vi "Current Loop 9505 (FPGA).vi"() -> ()   [LabVIEW 2011]
uses:
  <vilib>/LabVIEW Targets/FPGA/cRIO/cRIO-9505/controls.llb/_nicrio_cRIO-9505_DriveStatus.ctl
  <vilib>/Platform/TimedLoop/XDataNode/timing_clust.ctl
  <vilib>/Platform/TimedLoop/XDataNode/nitl_modes.ctl
  <vilib>/Platform/TimedLoop/XDataNode/wakeup.ctl
  <vilib>/LabVIEW Targets/FPGA/cRIO/cRIO-9505/controls.llb/_nicrio_cRIO-9505_DriveDirection.ctl
  <vilib>/rvi/eio/common/nirviEmuTemplateMethod_errors.vi
  <vilib>/rvi/eio/common/nirviEmuTemplatePropertyGet_noerrors.vi
  <vilib>/Platform/TimedLoop/XDataNode/XDataNode.xnode
  <vilib>/eio/EIONode/EIONode.xnode
  <vilib>/eio/EIOMethodNode/EIOMethodNode.xnode
  <vilib>/eio/EIOPropertyNode/EIOPropertyNode.xnode
  <vilib>/Platform/TimedLoop/XDataNode/XDNodeRunTimeDep.lvlib
  <vilib>/rvi/eio/common/nirviEmuTemplatePropertyGet_errors.vi
  <vilib>/rvi/eio/common/nirviEmuTemplatePropertySet_errors.vi
  <vilib>/rvi/eio/common/nirviEmuTemplatePropertySet_noerrors.vi
panel:
  out "Sample Current Loop Counter 2 i":i32(graph)
  out "Sample Current Loop Counter 1 i":i32(graph)
  out "PWM Loop Counter 2 i":i32(graph)
  out "PWM Loop Counter 1 i":i32(graph)
  out "Current Loop Counter 1 i":i32(graph)
  out "Current Loop Counter 2 i":i32(graph)
  out "Waveform Chart 4":i16(graph)
  out "Waveform Chart 3":i16(graph)
  out "Waveform Chart 2":i16(graph)
  in  "Trig AI 2":bool
  in  "Current PI gains 2":T1={"Proportional Gain"=20, "Integral Gain"=10, "Derivative Gain"=0}
  in  "Current Feedback 2":i16
  in  "Current Limit 2":i16 caption="Setpoint"
  in  "Current Setpoint 2":i16 caption="Setpoint"
  in  "Current Loop\nRate (usec) 2":u32=50
  out "PWM Duty Cycle 2":i16
  out "Vsup Present 2":bool
  out "Drive Fault 2":bool
  out "Drive Status 2":T2
  out "Temp Fault 2":bool
  in  "Enable\nDrive 2":bool
  in  "Disable\nDrive 2":bool
  out "Waveform Chart":i16(graph)
  in  "Trig AI":bool
  out "Vsup Present":bool
  out "Drive Fault":bool
  out "Drive Status":T2
  out "Temp Fault":bool
  in  "Enable\nDrive":bool
  in  "Disable\nDrive":bool
  in  "Current PI gains":T1={"Proportional Gain"=20, "Integral Gain"=10, "Derivative Gain"=0}
  in  "Current Feedback":i16
  in  "Current Limit":i16 caption="Setpoint"
  in  "Current Setpoint":i16 caption="Setpoint"
  in  "Current Loop\nRate (usec)":u32=50
  out "PWM Duty Cycle":i16
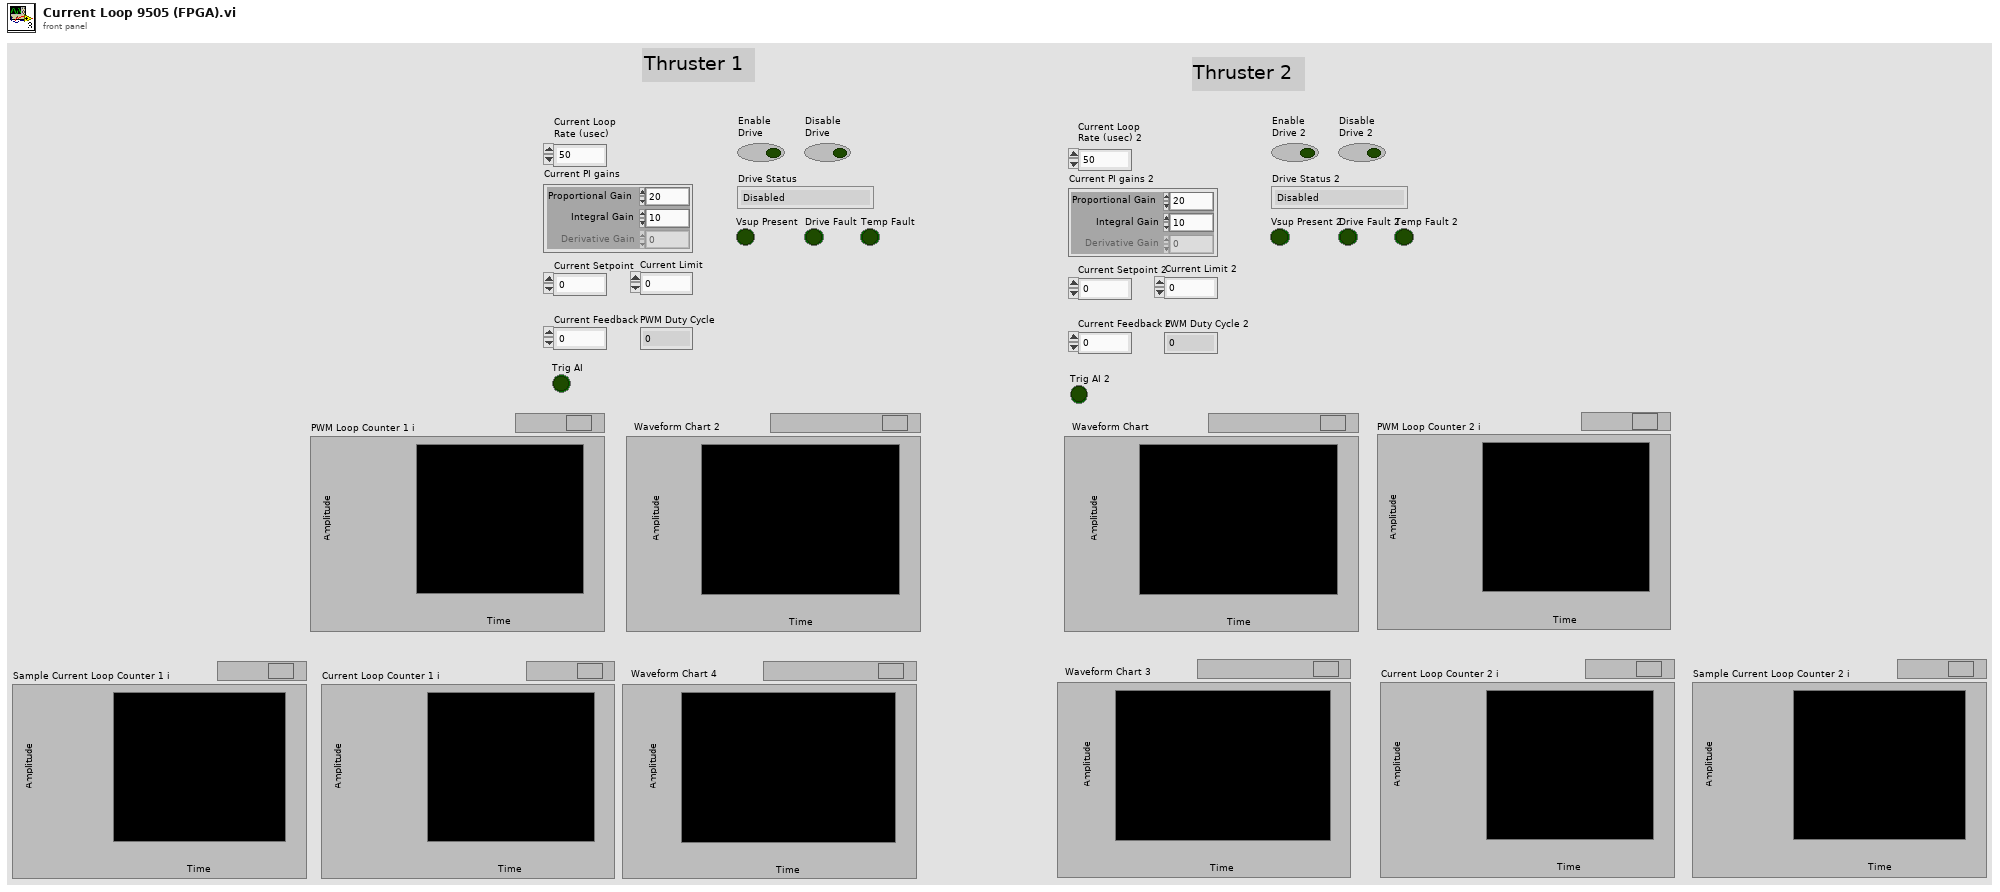
[diagram p1: front panel]
types:
  T1 = cluster{"Proportional Gain":i16, "Integral Gain":i16, "Derivative Gain":i16}
  T2 = typedef "_nicrio_cRIO-9505_DriveStatus.ctl" = enum8{"Enabled", "Disabled", "Disabled by Drive Fault", "Disabled by Temp. Fault", "Disabled by E-Stop", "Unknown"}
  T3 = typedef "XDNodeRunTimeDep.lvlib/timing_clust.ctl" = cluster{"Expected End [f-1]":u64, "Actual End [f-1]":u64, "Finished Late? [f-1]":bool, "Expected End [i-1]":u64, "Actual End [i-1]":u64, "Finished Late? [i-1]":bool, "Expected Start [i]":u64, "Actual Start [i]":u64, "Expected Start [f]":u64, "Actual Start [f]":u64, "Source Name":string, "Structure Name":string, "Period":i64, "Deadline":i64, "Offset":i64, "Start":i64, "Priority":i32, "Timeout":i32, "Mode":T4, "Wakeup Reason":T5, "Error":errorcluster, "Source Type":string, "Secondary Source Type":string, "Global End Time":u64, "Global Start Time":u64, "Frame Duration":u64, "Iteration Duration":u64, "Assigned CPU":i32, "I/O Scan Engine Mode":u32}
  T4 = typedef "XDNodeRunTimeDep.lvlib/nitl_modes.ctl" = enum32{"No Change", "Process missed periods, maintain original phase", "Discard missed periods, maintain original phase", "Process missed periods, ignore original phase", "Discard missed periods, ignore original phase"}
  T5 = typedef "XDNodeRunTimeDep.lvlib/wakeup.ctl" = enum32{"Normal", "Aborted", "Asynchronous wakeup", "Timing source error", "Timed loop error", "Timeout"}
  T6 = typedef "_nicrio_cRIO-9505_DriveDirection.ctl" = enum8{"Clockwise", "Counterclockwise"}
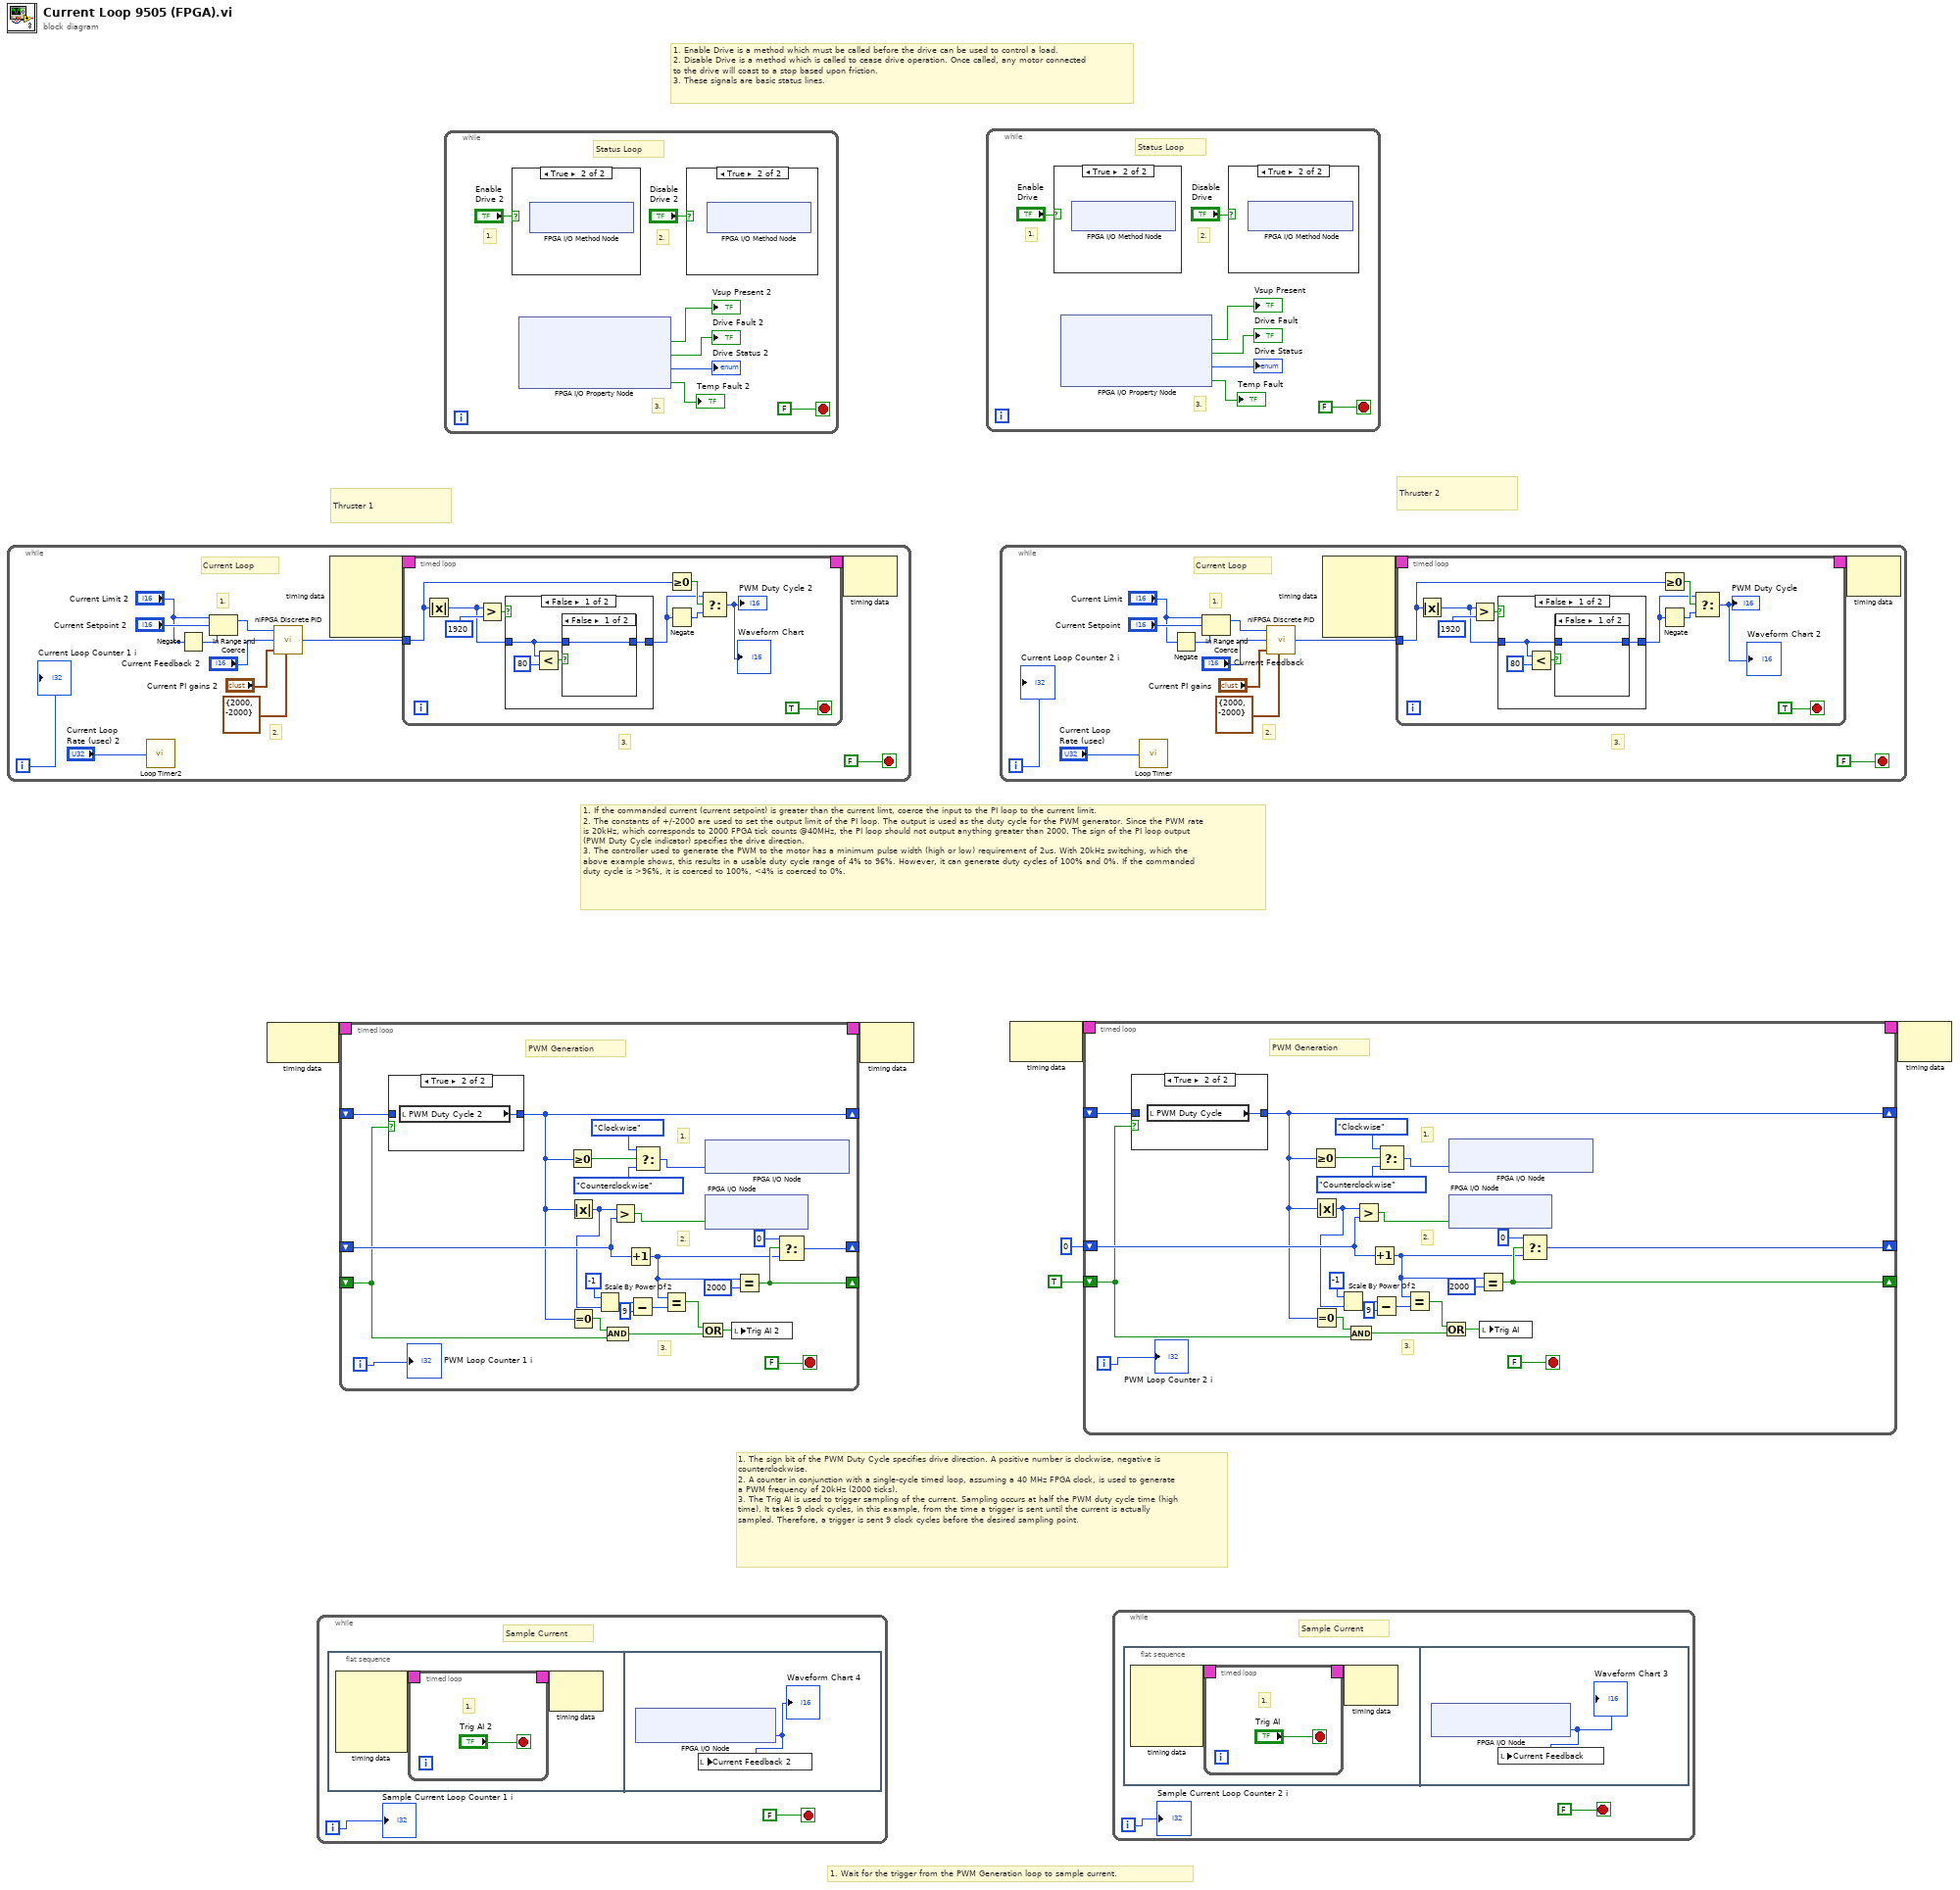
[diagram p0: block diagram]
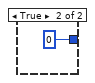
[diagram p3: hidden frame]
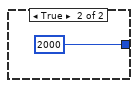
[diagram p4: hidden frame]
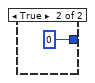
[diagram p10: hidden frame]
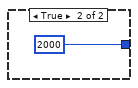
[diagram p11: hidden frame]
diagram:
  # "1. If the commanded current (current setpoint) is greater than the current limt, coerce the input to the PI loop to the current limit.\n2. The constants of +/-2000 are used to set the output limit of the PI loop. The output is used as the duty cycle for the PWM generator. Since the PWM rate is 20kHz, which corresponds to 2000 FPGA tick counts @40MHz, the PI loop should not output anything greater than 2000. The sign of the PI loop output (PWM Duty Cycle indicator) specifies the drive direction.\n3. The controller used to generate the PWM to the motor has a minimum pulse width (high or low) requirement of 2us. With 20kHz switching, which the above example shows, this results in a usable duty cycle range of 4% to 96%. However, it can generate duty cycles of 100% and 0%. If the commanded duty c..."
  # "Thruster 2"
  # "Thruster 1"
  # "1. Enable Drive is a method which must be called before the drive can be used to control a load.\n2. Disable Drive is a method which is called to cease drive operation. Once called, any motor connected to the drive will coast to a stop based upon friction.\n3. These signals are basic status lines."
  # "1. Wait for the trigger from the PWM Generation loop to sample current."
  # "1. The sign bit of the PWM Duty Cycle specifies drive direction. A positive number is clockwise, negative is counterclockwise.\n2. A counter in conjunction with a single-cycle timed loop, assuming a 40 MHz FPGA clock, is used to generate a PWM frequency of 20kHz (2000 ticks).\n3. The Trig AI is used to trigger sampling of the current. Sampling occurs at half the PWM duty cycle time (high time). It takes 9 clock cycles, in this example, from the time a trigger is sent until the current is actually sampled. Therefore, a trigger is sent 9 clock cycles before the desired sampling point."
  n1 = while {
    i -> [w7]
    stop <- FALSE stop-if-true
    # "3."
    # "2."
    # "1."
    # "Current Loop"
    n2 = call "Loop Timer2"("Count(uSec)"="Current Loop\nRate (usec) 2") -> ()  [unwired: 1 out]
    n3 = Negate(x="Current Limit 2") -> (-x=w12:i16)
    n4 = In Range and Coerce(upper limit="Current Limit 2", x="Current Setpoint 2", lower limit=w12) -> (coerced(x)=w10:i16)  [unwired: 1 out]
    n5 = call <vilib>:"niFPGA Discrete PID.vi"("setpoint"=w10, "process variable"="Current Feedback 2", "PID gains (x 2^8)"="Current PI gains 2", "output range"=cluster{"output high":i16, "output low":i16} {"output high"=2000, "output low"=-2000}) -> ("output"=w16:i16)  [unwired: 1 in, 4 out]
    n6 = node-c288() -> (w15:T3)  [unwired: 4 out]
    n7 = timed-loop {
      timing: w15 -> [_]
      timing-out: [_] -> w14
      tunnel: w16 -> [w22]
      stop <- TRUE stop-if-true
      n8 = Absolute Value(x=w22) -> (abs(x)=w23:i16)
      n9 = Greater?(x=w23, y=i16 1920) -> (0:w25:bool)
      n10 = case shown="False" w25 {
        tunnel: [w31 i16 2000] -> w24
        tunnel: w23 -> [w29 _]
        frame False {
          n11 = Less?(x=w29, y=i16 80) -> (x < y?=w30:bool)
          n12 = case shown="False" w30 {
            tunnel: [w33 i16 0] -> w31
            tunnel: w29 -> [w33 _]
            frame False {
            }
            frame True {
            }
          }
        }
        frame True {
        }
      }
      n13 = Greater Or Equal To 0?(x=w22) -> (x >= 0?=w28:bool)
      n14 = Negate(x=w24) -> (-x=w27:i16)
      n15 = Select(t=w24, s=w28, f=w27) -> (s? t:f=→"PWM Duty Cycle 2" →"Waveform Chart":i16)
    }
    n16 = node-c288(w14) -> ()  [unwired: 1 out]
    "Current Loop Counter 1 i" <- w7
  }
  n17 = node-c288() -> (w2:T3)  [unwired: 1 out]
  n18 = while {
    i -> [w40]
    stop <- FALSE stop-if-true
    # "Sample Current"
    n19 = flat-sequence {
      frame #0 {
        n20 = node-c288() -> (w43:T3)  [unwired: 4 out]
        n21 = timed-loop {
          timing: w43 -> [_]
          timing-out: [_] -> w42
          stop <- "Trig AI 2" stop-if-true
          # "1."
        }
        n22 = node-c288(w42) -> ()  [unwired: 1 out]
      }
      frame #1 {
        n23 = xnode "FPGA I/O Node"() -> ("Mod2/Current Sense"=w49:i16)  [unwired: 1 in, 1 out]
        "Waveform Chart 4" <- w49
        n24 = local write "Current Feedback 2"(w49) -> ()
      }
    }
    "Sample Current Loop Counter 1 i" <- w40
  }
  n25 = timed-loop {
    timing: w2 -> [_]
    timing-out: [_] -> w1
    shift-right: [w71] -> _
    shift-left: _ -> [w74]
    shift-right: [w70] -> _
    shift-left: _ -> [w67]
    shift-right: [w56] -> _
    shift-left: _ -> [w69]
    i -> [w50]
    stop <- FALSE stop-if-true
    # "3."
    # "2."
    # "1."
    # "PWM Generation"
    n26 = case shown="True" w67 {
      tunnel: [w75 w76] -> w56
      tunnel: w69 -> [w75 _]
      frame False {
      }
      frame True {
        n27 = local read "PWM Duty Cycle 2"() -> (w76:i16)
      }
    }
    n28 = Greater Or Equal To 0?(x=w56) -> (x >= 0?=w63:bool)
    n29 = Absolute Value(x=w56) -> (abs(x)=w54:i16)
    n30 = Equal To 0?(x=w56) -> (x = 0?=w68:bool)
    n31 = Scale By Power Of 2(n=i8 -1, x=w54) -> (x*2^n=w58:i16)
    n32 = And(x=w68, y=w67) -> (x .and. y?=w64:bool)
    n33 = Greater?(x=w54, y=w74) -> (0:w51:bool)
    n34 = Increment(x=w74) -> (x+1=w66:i16)
    n35 = Subtract(x=w58, y=i8 9) -> (x-y=w57:i16)
    n36 = Select(t=_nicrio_cRIO-9505_DriveDirection."Clockwise", s=w63, f=_nicrio_cRIO-9505_DriveDirection."Counterclockwise") -> (s? t:f=w52:T6)
    n37 = Equal?(x=w66, y=w57) -> (x = y?=w65:bool)
    n38 = Or(x=w65, y=w64) -> (x .or. y?=w60:bool)
    n39 = xnode "FPGA I/O Node"("Mod2/Drive Direction"=w52) -> ()  [unwired: 1 in, 1 out]
    n40 = xnode "FPGA I/O Node"("Mod2/Motor"=w51) -> ()  [unwired: 1 in, 1 out]
    n41 = local write "Trig AI 2"(w60) -> ()
    n42 = Equal?(x=w66, y=i16 2000) -> (x = y?=w70:bool)
    n43 = Select(t=i16 0, s=w70, f=w66) -> (s? t:f=w71:i16)
    "PWM Loop Counter 1 i" <- w50
  }
  n44 = while {
    stop <- FALSE stop-if-true
    # "3."
    # "2."
    # "1."
    # "Status Loop"
    n45 = case shown="True" "Enable\nDrive 2" {
      frame False {
      }
      frame True {
        n46 = xnode "FPGA I/O Method Node"() -> ()  [unwired: 1 in, 1 out]
      }
    }
    n47 = xnode "FPGA I/O Property Node"() -> ("Vsup Present"=→"Vsup Present 2":bool, "Drive Fault"=→"Drive Fault 2":bool, "Drive Status"=→"Drive Status 2":T2, "Over Temperature Fault"=→"Temp Fault 2":bool)  [unwired: 1 in, 1 out]
    n48 = case shown="True" "Disable\nDrive 2" {
      frame False {
      }
      frame True {
        n49 = xnode "FPGA I/O Method Node"() -> ()  [unwired: 1 in, 1 out]
      }
    }
  }
  n50 = node-c288(w1) -> ()  [unwired: 1 out]
  n51 = while {
    stop <- FALSE stop-if-true
    # "3."
    # "2."
    # "1."
    # "Status Loop"
    n52 = case shown="True" "Enable\nDrive" {
      frame False {
      }
      frame True {
        n53 = xnode "FPGA I/O Method Node"() -> ()  [unwired: 1 in, 1 out]
      }
    }
    n54 = xnode "FPGA I/O Property Node"() -> ("Vsup Present"=→"Vsup Present":bool, "Drive Fault"=→"Drive Fault":bool, "Drive Status"=→"Drive Status":T2, "Over Temperature Fault"=→"Temp Fault":bool)  [unwired: 1 in, 1 out]
    n55 = case shown="True" "Disable\nDrive" {
      frame False {
      }
      frame True {
        n56 = xnode "FPGA I/O Method Node"() -> ()  [unwired: 1 in, 1 out]
      }
    }
  }
  n57 = while {
    i -> [w93]
    stop <- FALSE stop-if-true
    # "3."
    # "2."
    # "1."
    # "Current Loop"
    n58 = call "Loop Timer"("Count(uSec)"="Current Loop\nRate (usec)") -> ()  [unwired: 1 out]
    n59 = Negate(x="Current Limit") -> (-x=w98:i16)
    n60 = In Range and Coerce(upper limit="Current Limit", x="Current Setpoint", lower limit=w98) -> (coerced(x)=w96:i16)  [unwired: 1 out]
    n61 = call <vilib>:"niFPGA Discrete PID.vi"("setpoint"=w96, "process variable"="Current Feedback", "PID gains (x 2^8)"="Current PI gains", "output range"=cluster{"output high":i16, "output low":i16} {"output high"=2000, "output low"=-2000}) -> ("output"=w102:i16)  [unwired: 1 in, 4 out]
    n62 = node-c288() -> (w101:T3)  [unwired: 4 out]
    n63 = timed-loop {
      timing: w101 -> [_]
      timing-out: [_] -> w100
      tunnel: w102 -> [w108]
      stop <- TRUE stop-if-true
      n64 = Absolute Value(x=w108) -> (abs(x)=w109:i16)
      n65 = Greater?(x=w109, y=i16 1920) -> (0:w111:bool)
      n66 = case shown="False" w111 {
        tunnel: [w117 i16 2000] -> w110
        tunnel: w109 -> [w115 _]
        frame False {
          n67 = Less?(x=w115, y=i16 80) -> (x < y?=w116:bool)
          n68 = case shown="False" w116 {
            tunnel: [w119 i16 0] -> w117
            tunnel: w115 -> [w119 _]
            frame False {
            }
            frame True {
            }
          }
        }
        frame True {
        }
      }
      n69 = Greater Or Equal To 0?(x=w108) -> (x >= 0?=w114:bool)
      n70 = Negate(x=w110) -> (-x=w113:i16)
      n71 = Select(t=w110, s=w114, f=w113) -> (s? t:f=→"PWM Duty Cycle" →"Waveform Chart 2":i16)
    }
    n72 = node-c288(w100) -> ()  [unwired: 1 out]
    "Current Loop Counter 2 i" <- w93
  }
  n73 = node-c288() -> (w6:T3)  [unwired: 1 out]
  n74 = timed-loop {
    timing: w6 -> [_]
    timing-out: [_] -> w5
    shift-right: [w147] -> _
    shift-left: i16 0 -> [w150]
    shift-right: [w146] -> _
    shift-left: TRUE -> [w143]
    shift-right: [w132] -> _
    shift-left: _ -> [w145]
    i -> [w126]
    stop <- FALSE stop-if-true
    # "3."
    # "2."
    # "1."
    # "PWM Generation"
    n75 = case shown="True" w143 {
      tunnel: [w151 w152] -> w132
      tunnel: w145 -> [w151 _]
      frame False {
      }
      frame True {
        n76 = local read "PWM Duty Cycle"() -> (w152:i16)
      }
    }
    n77 = Greater Or Equal To 0?(x=w132) -> (x >= 0?=w139:bool)
    n78 = Absolute Value(x=w132) -> (abs(x)=w130:i16)
    n79 = Equal To 0?(x=w132) -> (x = 0?=w144:bool)
    n80 = Scale By Power Of 2(n=i8 -1, x=w130) -> (x*2^n=w134:i16)
    n81 = And(x=w144, y=w143) -> (x .and. y?=w140:bool)
    n82 = Greater?(x=w130, y=w150) -> (0:w127:bool)
    n83 = Increment(x=w150) -> (x+1=w142:i16)
    n84 = Subtract(x=w134, y=i8 9) -> (x-y=w133:i16)
    n85 = Select(t=_nicrio_cRIO-9505_DriveDirection."Clockwise", s=w139, f=_nicrio_cRIO-9505_DriveDirection."Counterclockwise") -> (s? t:f=w128:T6)
    n86 = Equal?(x=w142, y=w133) -> (x = y?=w141:bool)
    n87 = Or(x=w141, y=w140) -> (x .or. y?=w136:bool)
    n88 = xnode "FPGA I/O Node"("Mod4/Drive Direction"=w128) -> ()  [unwired: 1 in, 1 out]
    n89 = xnode "FPGA I/O Node"("Mod4/Motor"=w127) -> ()  [unwired: 1 in, 1 out]
    n90 = Equal?(x=w142, y=i16 2000) -> (x = y?=w146:bool)
    n91 = local write "Trig AI"(w136) -> ()
    n92 = Select(t=i16 0, s=w146, f=w142) -> (s? t:f=w147:i16)
    "PWM Loop Counter 2 i" <- w126
  }
  n93 = while {
    i -> [w155]
    stop <- FALSE stop-if-true
    # "Sample Current"
    n94 = flat-sequence {
      frame #0 {
        n95 = node-c288() -> (w158:T3)  [unwired: 4 out]
        n96 = timed-loop {
          timing: w158 -> [_]
          timing-out: [_] -> w157
          stop <- "Trig AI" stop-if-true
          # "1."
        }
        n97 = node-c288(w157) -> ()  [unwired: 1 out]
      }
      frame #1 {
        n98 = xnode "FPGA I/O Node"() -> ("Mod4/Current Sense"=w164:i16)  [unwired: 1 in, 1 out]
        "Waveform Chart 3" <- w164
        n99 = local write "Current Feedback"(w164) -> ()
      }
    }
    "Sample Current Loop Counter 2 i" <- w155
  }
  n100 = node-c288(w5) -> ()  [unwired: 1 out]
